vi "BH Druck  PACE Series Sense Pressures with Barometer.vi.vi"() -> ()   [LabVIEW 2022 SP3]
uses:
  <vilib>/Utility/error.llb/DialogType.ctl
  BH Druck PACE Series.lvclass
panel:
  out "-ve Source /mbar":dbl format="%#.10g"
  out "+ve Source /mbar":dbl format="%#.10g"
  out "Measured Pressure /mbar":dbl format="%#.10g"
  out "-FS range/mbar":dbl
  out "+FS range/mbar":dbl
  out "Read Unit":string
  out "-ve Source":dbl format="%#.10g"
  out "+ve Source":dbl format="%#.10g"
  out "Measured Pressure":dbl format="%#.10g"
  out "Range":string
  out "-FS range":dbl
  out "+FS range":dbl
  in  "Unit (mbar)":u16(ring) items=["mbar", "bar", "Pa", "hPa", "kPa", "mPa", "mmHg@0°C", "cmHg@0°C", "mHg@0°C", "inHg@0°C", "kg/cm2", "kg/m2", "mmH2O@4°C", "cmH2O@4°C", "mH2O@4°C", "mmH2O@20°C", "cmH2O@20°C", "mH2O@20°C", "torr", "atm", "psi", "lb/ft2", "inH2O@4°C", "inH2O@20°C", "inH2O@60°F", "ftH2O@4°C", "ftH2O@20°C", "ftH2O@60°F", "UserUnit1", "UserUnit2", "UserUnit3", "UserUnit4"]
  in  "Channel (0: Channel A)":enum16{"Channel A", "Channel B"}(ring)
  in  "VISA resource name":refnum<visa-resource-name>
  # "(c)2010-2020  BH  Druck Ltd.  ALL RIGHTS RESERVED."
  # "Setup instrument"
  # "Read from instrument in current unit"
  # "Convert to mbar unit to check unit convert ratio"
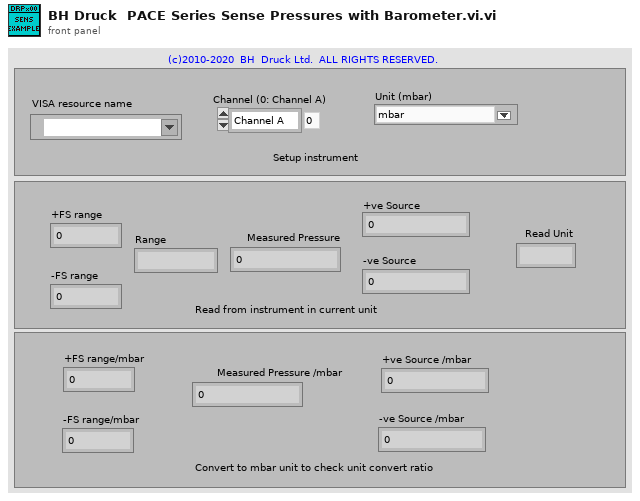
[diagram p1: front panel]
types:
  T1 = typedef "DialogType.ctl" = u16
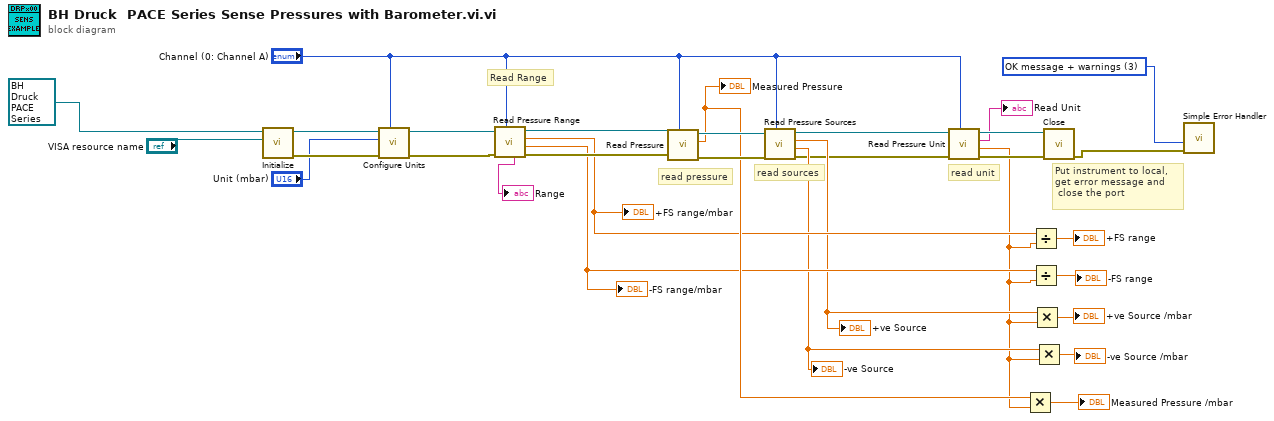
[diagram p0: block diagram]
diagram:
  w10 = T1 3 items=["no dialog", "OK message", "continue or stop message", "OK message + warnings", "continue/stop + warnings"] ("type of dialog (OK msg:1)")
  # "Read Range"
  # "read pressure"
  # "read sources"
  # "read unit"
  # "Put instrument to local, \nget error message and\n close the port"
  n1 = call-dynamic "Initialize.vi"("VISA resource name"="VISA resource name", "BH Druck PACE Series in"=refnum<class "BH Druck PACE Series.lvclass"> refnum) -> ("error out"=w12:errorcluster, "BH Druck PACE Series out"=w13:refnum<class "BH Druck PACE Series.lvclass">)  [unwired: 7 in]
  n2 = call-dynamic "Configure Units.vi"("Channel (0: Channel A)"="Channel (0: Channel A)", "error in (no error)"=w12, "Unit (mbar)"="Unit (mbar)", "BH Druck PACE Series in"=w13) -> ("error out"=w3:errorcluster, "BH Druck PACE Series out"=w4:refnum<class "BH Druck PACE Series.lvclass">)  [unwired: 6 in]
  n3 = call-dynamic "Read Pressure Range.vi"("Channel (0: Channel A)"="Channel (0: Channel A)", "error in (no error)"=w3, "BH Druck PACE Series in"=w4) -> ("error out"=w25:errorcluster, "-FS Range/mbar"=w21:dbl, "+FS Range/mbar"=w22:dbl, "BH Druck PACE Series out"=w26:refnum<class "BH Druck PACE Series.lvclass">, "Range"=→"Range":string)  [unwired: 4 in]
  "+FS range/mbar" <- w22
  "-FS range/mbar" <- w21
  n4 = call-dynamic "Read Pressure.vi"("Channel (0: Channel A)"="Channel (0: Channel A)", "error in (no error)"=w25, "BH Druck PACE Series in"=w26) -> ("error out"=w30:errorcluster, "Measured Pressure"=w24:dbl, "BH Druck PACE Series out"=w31:refnum<class "BH Druck PACE Series.lvclass">)  [unwired: 6 in]
  "Measured Pressure" <- w24
  n5 = call-dynamic "Read Pressure Sources.vi"("Channel (0: Channel A)"="Channel (0: Channel A)", "error in (no error)"=w30, "BH Druck PACE Series in"=w31) -> ("error out"=w6:errorcluster, "Vacuum Sensor -ve Source"=w20:dbl, "Pressure Sensor  +ve Source"=w19:dbl, "BH Druck PACE Series out"=w5:refnum<class "BH Druck PACE Series.lvclass">)  [unwired: 5 in]
  "+ve Source" <- w19
  "-ve Source" <- w20
  n6 = call-dynamic "Read Pressure Unit.vi"("Channel (0: Channel A)"="Channel (0: Channel A)", "error in (no error)"=w6, "BH Druck PACE Series in"=w5) -> ("error out"=w28:errorcluster, "Unit Convert"=w18:dbl, "Selected Unit"=→"Read Unit":string, "BH Druck PACE Series out"=w29:refnum<class "BH Druck PACE Series.lvclass">)  [unwired: 5 in]
  n7 = Multiply(x=w24, y=w18) -> (x*y=→"Measured Pressure /mbar":dbl)
  n8 = Divide(x=w22, y=w18) -> (x/y=→"+FS range":dbl)
  n9 = Divide(x=w21, y=w18) -> (x/y=→"-FS range":dbl)
  n10 = Multiply(x=w19, y=w18) -> (x*y=→"+ve Source /mbar":dbl)
  n11 = Multiply(x=w20, y=w18) -> (x*y=→"-ve Source /mbar":dbl)
  n12 = call "Close.vi"("error in (no error)"=w28, "BH Druck PACE Series in"=w29) -> ("error out"=w11:errorcluster)  [unwired: 8 in, 1 out]
  n13 = call <vilib>:"Simple Error Handler.vi"("type of dialog (OK msg:1)"=w10, "error in (no error)"=w11) -> ()  [unwired: 3 in, 5 out]
